vi "SetdBBase.vi"(8 "错误输入（无错误）":errorcluster, 10 "增益值索引":u16) -> (0 "错误输出":errorcluster)   [LabVIEW 2018]
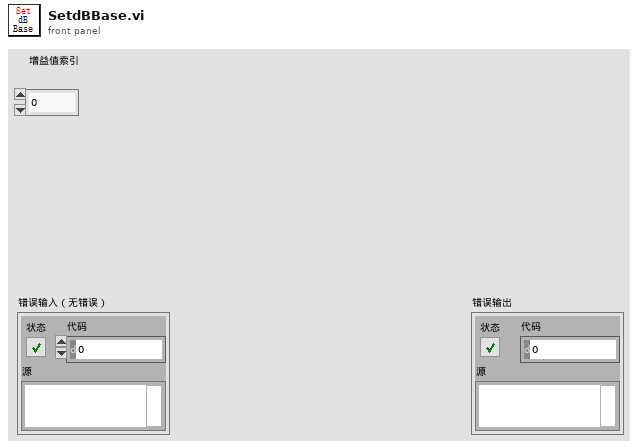
[diagram p1: front panel]
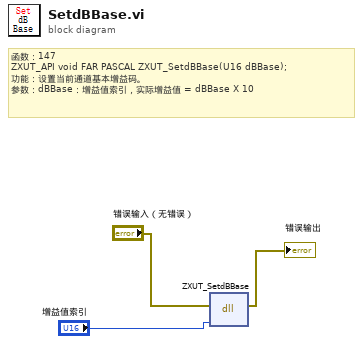
[diagram p0: block diagram]
diagram:
  # "函数：147\nZXUT_API void\tFAR PASCAL ZXUT_SetdBBase(U16 dBBase);\n功能：设置当前通道基本增益码。\n参数：dBBase：增益值索引，实际增益值 = dBBase X 10"
  n1 = dll-call lib="PTH2Rabs E软件项目超声超声子VI函数VI\tTCG处理ZXUTConfigMgr.dll" fn="ZXUT_SetdBBase"(error in="错误输入（无错误）", "dBBase"="增益值索引") -> (error out=→"错误输出":errorcluster)  [unwired: 4 in, 1 out]
